vi "configure.vi"(8 "error in (no error)":errorcluster, 11 "SignalReaderDL091205FPGA in":refnum<class "SignalReaderDL091205FPGA.lvclass">) -> (0 "error out":errorcluster, 3 "SignalReaderDL091205FPGA out":refnum<class "SignalReaderDL091205FPGA.lvclass">)   [LabVIEW 2010, in "SignalReaderDL091205FPGA.lvclass"]
doc: "The dynamic dispatch version of this VI loads and displays the configuration file associated with the plug-in object. The user modify and save the configuration data."
uses:
  SignalReaderDL091205FPGA.lvclass
  common/xcontrols/XComponentSpecification/XComponentSpecification/XComponentSpecification.xctl
  SignalReaderDL091205FPGA.lvclass/SignalReaderDL091205FPGA.ctl
  FPGAWrapper/GenericFPGAWrapper/GenericFPGAWrapper/GenericFPGAWrapper.lvclass
  common/classes/GenericComponent/GenericComponent/GenericComponent.lvclass
panel:
  in  "FPGAWrapper spec":T1(xcontrol)
  in  "time-out":dbl[unit]=0.5
  in  "Number of channels":i32=1 min=1
  out "LSID":string
  in  "cancelButton":bool
  in  "saveButton":bool
  out "Configuration":string
  # "Configure SignalReaderDL091205FPGA"
  # "FPGA wrapper"
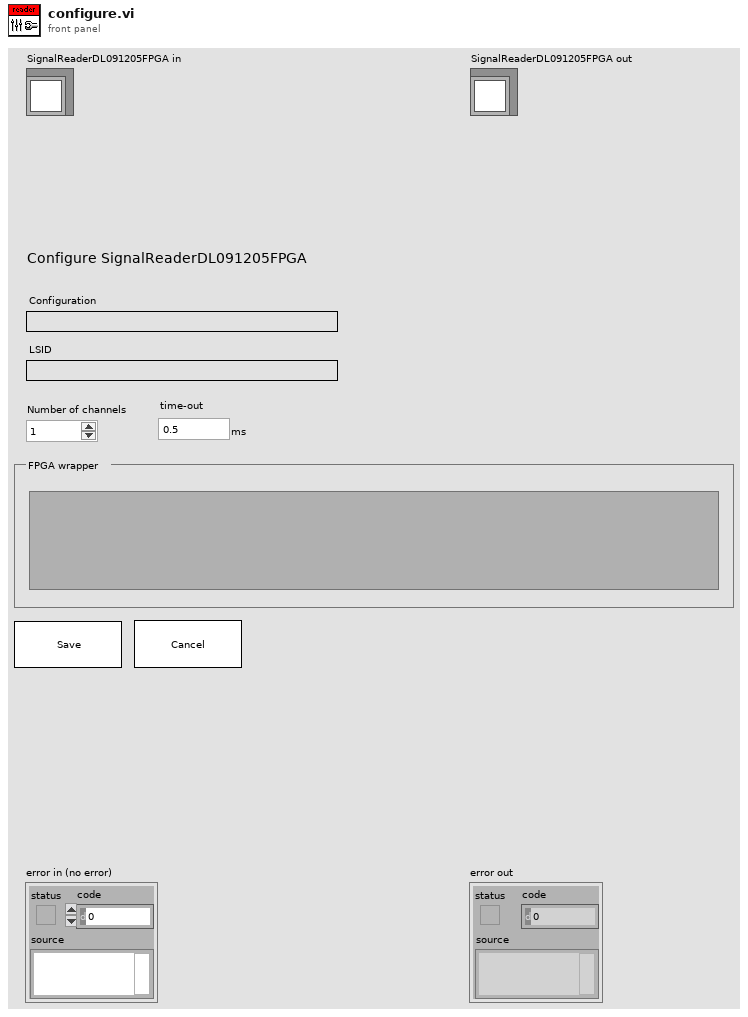
[diagram p1: front panel]
types:
  T1 = cluster{"class path":string, "configuration":string, "label":string, "settings name":string}
  T2 = typedef "plugin_specification.ctl" = cluster{"class path":string, "configuration":string, "label":string, "settings name":string}
  T3 = typedef "LSID_cluster.ctl" = cluster{"identifier":string, "revision":i32}
  T4 = typedef "SignalReaderDL091205FPGA.lvclass/config_data_cluster.ctl" = cluster{"FPGA wrapper":T2, "number of channels":i32, "LSID":T3, "time-out":dbl[unit]}
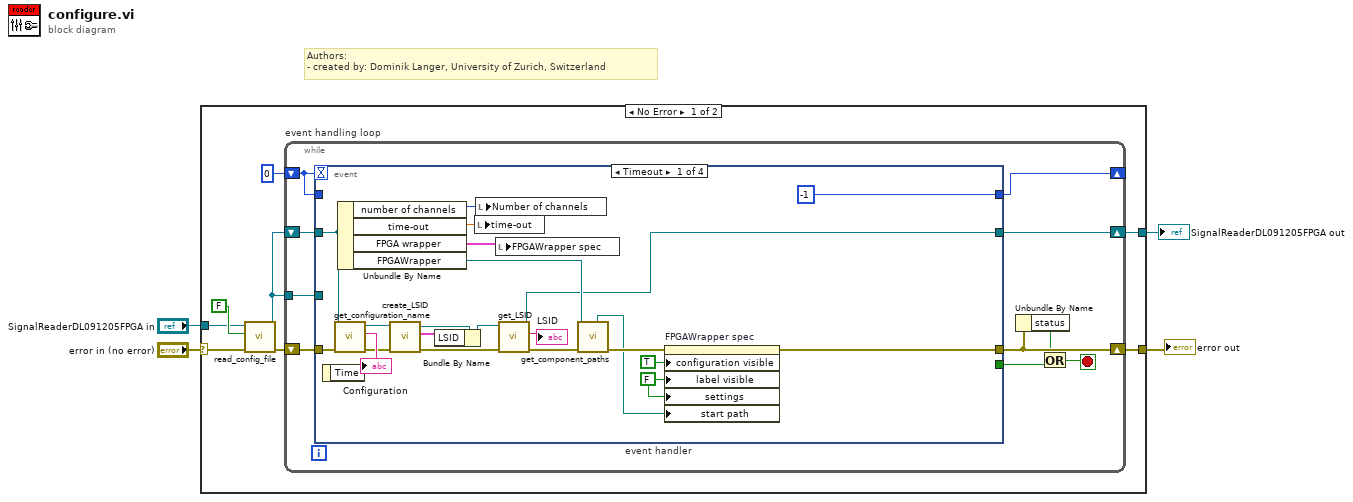
[diagram p0: block diagram]
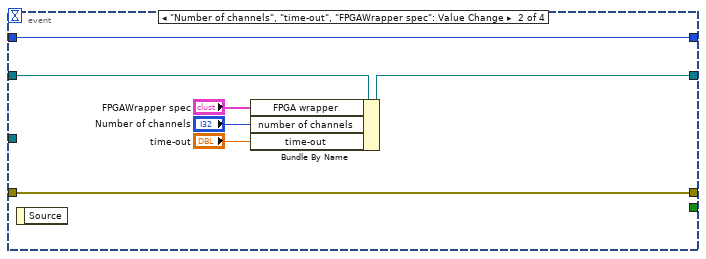
[diagram p2: hidden frame]
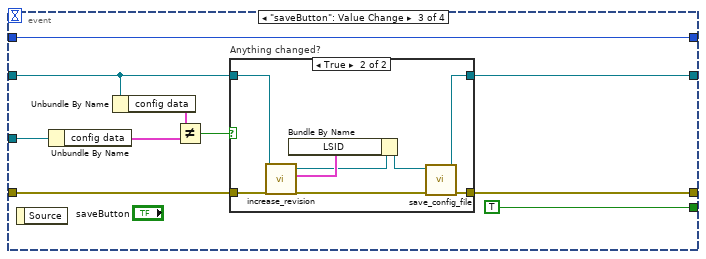
[diagram p3: hidden frame]
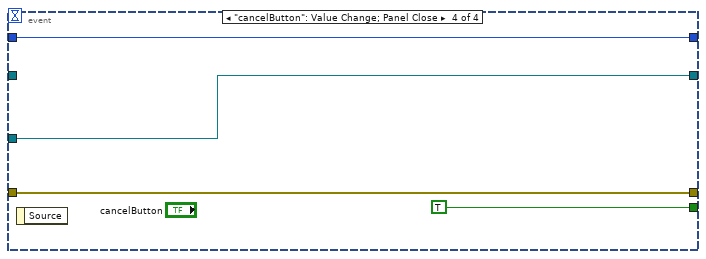
[diagram p5: hidden frame]
diagram:
  # "Authors: \n- created by: Dominik Langer, University of Zurich, Switzerland"
  n1 = case shown="No Error" "error in (no error)" {
    selector: "error in (no error)" -> [w11 w76]
    tunnel: "SignalReaderDL091205FPGA in" -> [w10 w77]
    tunnel: [w7 w77] -> w1
    tunnel: [w6 w76] -> w2
    frame No Error {
      n2 = call-dynamic "read_config_file.vi"("error in (no error)"=w11, "force load?"=FALSE, "GenericPlugin in"=w10) -> ("error out"=w9:errorcluster, "GenericPlugin out"=w5:refnum<class "SignalReaderDL091205FPGA.lvclass">)  [unwired: 7 out]
      n3 = while "event handling loop" {
        shift-right: [w16] -> w6
        shift-left: w9 -> [w22]
        shift-right: [w19] -> _
        shift-left: 0 -> [w20]
        shift-right: [w18] -> w7
        shift-left: w5 -> [w21]
        tunnel: w5 -> [w17]
        stop <- w13 stop-if-true
        n4 = event "event handler" shown="[0] Timeout" {
          selector: _ -> [_ _ _ _]
          dyn-events: _ -> [_ _ _ _]
          timeout: w20 -> [_ _ _ _]
          tunnel: w22 -> [w30 w45 w59 w74]
          tunnel: w21 -> [w33 w50 w55 _]
          tunnel: w20 -> [_ w51 w61 w75]
          tunnel: [-1 w51 w61 w75] -> w19
          tunnel: [w26 w45 w58 w74] -> w16
          tunnel: [w28 w47 w57 w72] -> w18
          tunnel: [_ _ TRUE TRUE] -> w15
          tunnel: w17 -> [_ _ w56 w72]
          event Timeout {
            w23 = FALSE ("label visible")
            n5 = event-data() -> ()  [unwired: 2 out]
            n6 = call "get_configuration_name.vi"("error in (no error)"=w30, "GenericPlugin.lvclass in"=w33) -> ("error out"=w42:errorcluster, "configuration name"=→"Configuration":string, "GenericPlugin.lvclass out"=w41:refnum<class "SignalReaderDL091205FPGA.lvclass">)  [unwired: 7 in]
            n7 = Unbundle By Name(w33) -> ("number of channels"=w34:i32, "time-out"=w35:dbl[unit], "FPGA wrapper"=w31:T2, "FPGAWrapper"=w29:refnum<class "GenericFPGAWrapper.lvclass">)
            n8 = call-dynamic "create_LSID.vi"("error in (no error)"=w42, "GenericPlugin in"=w41) -> ("error out"=w38:errorcluster, "current LSID"=w39:T3, "GenericPlugin out"=w40:refnum<class "SignalReaderDL091205FPGA.lvclass">)  [unwired: 7 in]
            n9 = Bundle By Name(cluster=w40, "LSID"=w39) -> (w36:refnum<class "SignalReaderDL091205FPGA.lvclass">)
            n10 = local write "time-out"(w35) -> ()
            n11 = local write "Number of channels"(w34) -> ()
            n12 = local write "FPGAWrapper spec"(w31) -> ()
            n13 = call-dynamic "get_LSID.vi"("error in (no error)"=w38, "GenericPlugin in"=w36) -> ("error out"=w32:errorcluster, "LSID (string)"=→"LSID":string, "GenericPlugin out"=w28:refnum<class "SignalReaderDL091205FPGA.lvclass">)  [unwired: 6 in, 1 out]
            n14 = call-dynamic "get_component_paths.vi"("error in (no error)"=w32, "GenericComponent in"=w29) -> ("error out"=w27:errorcluster, "component type directory"=w25:path)  [unwired: 4 in, 4 out]
            n15 = property on="FPGAWrapper spec" class="XComponentSpecification (strict"(error in=w27, "configuration visible"=TRUE, "label visible"=w23, "settings"=w23, "start path"=w25) -> (error out=w26:errorcluster)  [unwired: 1 in, 1 out]
          }
          event "Number of channels", "time-out", "FPGAWrapper spec": Value Change {
            n16 = event-data() -> ()  [unwired: 2 out]
            n17 = Bundle By Name(cluster=w50, "FPGA wrapper"="FPGAWrapper spec", "number of channels"="Number of channels", "time-out"="time-out") -> (w47:refnum<class "SignalReaderDL091205FPGA.lvclass">)
          }
          event "saveButton": Value Change {
            n18 = event-data() -> ()  [unwired: 2 out]
            n19 = Unbundle By Name(w56) -> ("config data"=w54:T4)
            n20 = Unbundle By Name(w55) -> ("config data"=w53:T4)
            n21 = Not Equal?(x=w53, y=w54) -> (x != y?=w52:bool)
            n22 = case "Anything changed?" shown="True" w52 {
              tunnel: w59 -> [w62 w69]
              tunnel: [w62 w71] -> w58
              tunnel: [w63 w70] -> w57
              tunnel: w55 -> [w63 w67]
              frame False {
              }
              frame True {
                n23 = call-dynamic "increase_revision.vi"("error in (no error)"=w69, "GenericPlugin in"=w67) -> ("error out"=w68:errorcluster, "new LSID"=w66:T3, "GenericPlugin out"=w65:refnum<class "SignalReaderDL091205FPGA.lvclass">)  [unwired: 7 in]
                n24 = Bundle By Name(cluster=w65, "LSID"=w66) -> (w64:refnum<class "SignalReaderDL091205FPGA.lvclass">)
                n25 = call-dynamic "save_config_file.vi"("error in (no error)"=w68, "GenericPlugin in"=w64) -> ("error out"=w71:errorcluster, "GenericPlugin out"=w70:refnum<class "SignalReaderDL091205FPGA.lvclass">)  [unwired: 2 in, 6 out]
              }
            }
          }
          event "cancelButton": Value Change; Panel Close {
            n26 = event-data() -> ()  [unwired: 2 out]
          }
        }
        n27 = Unbundle By Name(w16) -> ("status"=w14:bool)
        n28 = Or(x=w14, y=w15) -> (x .or. y?=w13:bool)
      }
    }
    frame Error {
    }
  }
  "error out" <- w2
  "SignalReaderDL091205FPGA out" <- w1
